vi "fullSpeed.vi"(10 "Throttle Buttons":bool[](array[boolean]), 11 "current motor value":dbl format="%#_13g") -> (3 "Output motor value":dbl format="%#_13g")   [LabVIEW 2018]
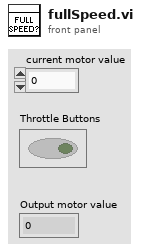
[diagram p1: front panel]
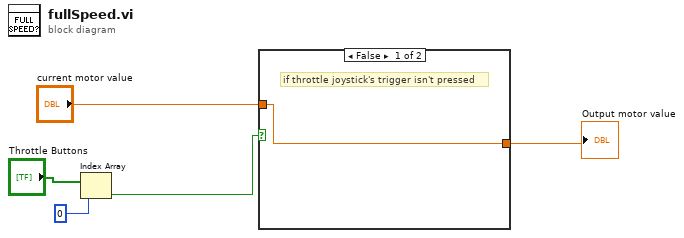
[diagram p0: block diagram]
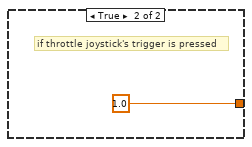
[diagram p2: hidden frame]
diagram:
  n1 = Index Array(array="Throttle Buttons", index=0) -> (element=w4:bool)
  n2 = case shown="False" w4 {
    tunnel: "current motor value" -> [w6 _]
    tunnel: [w6 1.0] -> w1
    frame False {
      # "if throttle joystick's trigger isn't pressed"
    }
    frame True {
      # "if throttle joystick's trigger is pressed"
    }
  }
  "Output motor value" <- w1
